vi "Measurement Logic.vi"(8 "error in":errorcluster, 9 "measurement configuration":T2={"TDMS File Location"="", "Run Action"="Create/Replace Wfm Group", "Wfm Group Name"="Wfm1", "Channel Names"=[], "Waveforms Summary JSON"=[]}, 10 "measure call context in":refnum<class "Measure Call Context.lvclass">) -> (0 "error out":errorcluster, 1 "measurement results":T1={"Final Waveform Group Name"="Empty"}, 2 "measure call context out":refnum<class "Measure Call Context.lvclass">)   [LabVIEW 2025, in "TDMS Waveform Creator.lvclass"]
doc: "Contains the core logic for executing the measurement."
uses:
  TDMS Waveform Creator.lvclass
  TDMS Waveform Creator.lvclass/TDMS Waveform Creator.ctl
  Measurement Results.ctl
  <vilib>/Plug-In SDKs/Measurements/Measure Call Context/Measure Call Context.lvclass
  Measurement Configuration.ctl
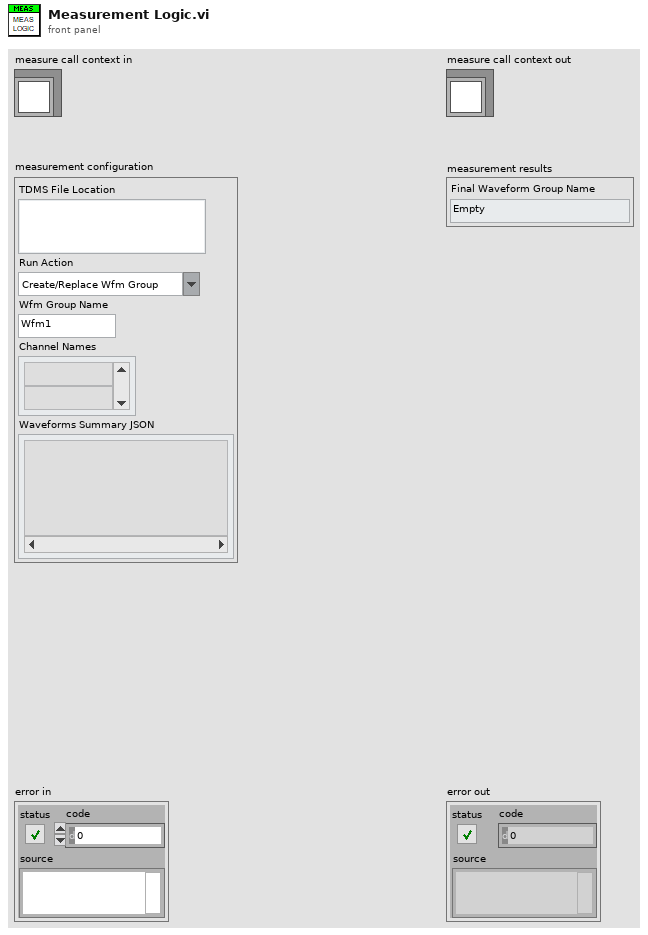
[diagram p1: front panel]
types:
  T1 = typedef "TDMS Waveform Creator.lvclass/Measurement Results.ctl" = cluster{"Final Waveform Group Name":string}
  T2 = typedef "TDMS Waveform Creator.lvclass/Measurement Configuration.ctl" = cluster{"TDMS File Location":string, "Run Action":string, "Wfm Group Name":string, "Channel Names":string[], "Waveforms Summary JSON":string[]}
  T3 = typedef "Event Messenger-bool.lvlib/))Channel.ctl" = refnum<queue>
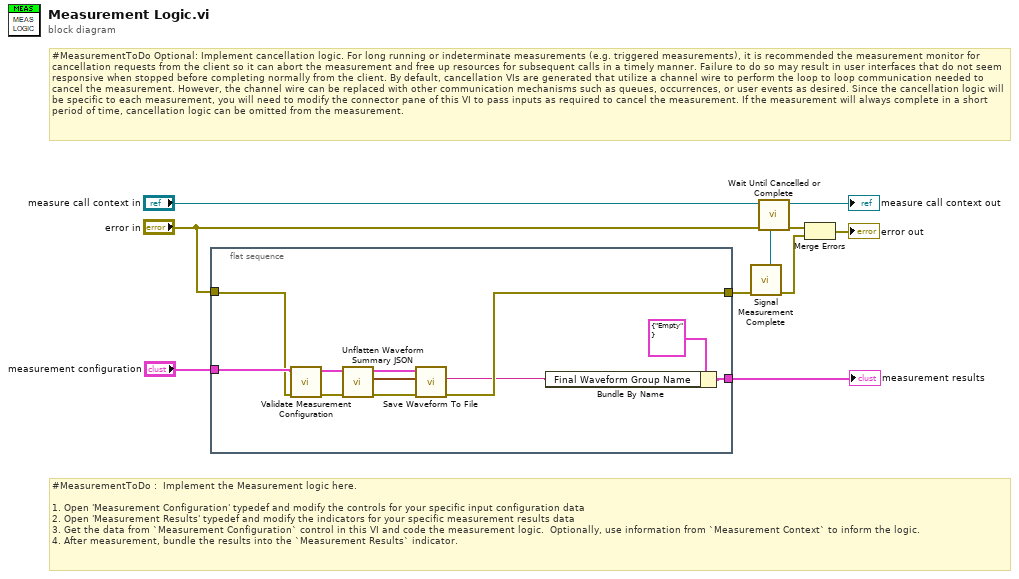
[diagram p0: block diagram]
diagram:
  # "#MeasurementToDo Optional: Implement cancellation logic. For long running or indeterminate measurements (e.g. triggered measurements), it is recommended the measurement monitor for cancellation requests from the client so it can abort the measurement and free up resources for subsequent calls in a timely manner. Failure to do so may result in user interfaces that do not seem responsive when stopped before completing normally from the client. By default, cancellation VIs are generated that utilize a channel wire to perform the loop to loop communication needed to cancel the measurement. However, the channel wire can be replaced with other communication mechanisms such as queues, occurrences, or user events as desired. Since the cancellation logic will be specific to each measurement, you will need to modify the connector pane of this VI to pass inputs as required to cancel the measurement. If the measurement will always complete in a short period of time, cancellation logic can be omitted from the measurement."
  # "#MeasurementToDo :  Implement the Measurement logic here.\n\n1. Open 'Measurement Configuration' typedef and modify the controls for your specific input configuration data\n2. Open 'Measurement Results' typedef and modify the indicators for your specific measurement results data\n3. Get the data from `Measurement Configuration` control in this VI and code the measurement logic.  Optionally, use information from `Measurement Context` to inform the logic.\n4. After measurement, bundle the results into the `Measurement Results` indicator."
  n1 = flat-sequence {
    tunnel: "measurement configuration" -> [w19]
    tunnel: [w20] -> w9
    tunnel: "error in" -> [w17]
    tunnel: [w14] -> w5
    frame #0 {
      n2 = call "Validate Measurement Configuration.vi"("error in"=w17, "Measurement Configuration In"=w19) -> ("error out"=w18:errorcluster, "Measurement Configuration Out"=w15:T2)  [unwired: 8 in]
      n3 = call "Unflatten Waveform Summary JSON.vi"("error in"=w18, "Measurement Configuration In"=w15) -> ("error out"=w16:errorcluster, "Waveforms"=w11:waveform(dbl)[], "Measurement Configuration Out"=w13:T2)  [unwired: 7 in]
      n4 = call "Save Waveform To File.vi"("error in"=w16, "Waveforms"=w11, "Measurement Configuration In"=w13) -> ("error out"=w14:errorcluster, "Final Wfm Group Name"=w12:string)  [unwired: 6 in, 1 out]
      n5 = Bundle By Name(cluster=T1 {"Final Waveform Group Name"="Empty"} ("Measurement Results"), "Final Waveform Group Name"=w12) -> (w20:T1)
    }
  }
  n6 = call "Signal Measurement Complete.vi"("error in (no error)"=w5) -> ("error out"=w3:errorcluster, "done channel"=w4:T3)  [unwired: 9 in]
  n7 = call "Wait Until Cancelled or Complete.vi"("done channel"=w4, "error in (no error)"="error in", "measure call context in"="measure call context in") -> ("error out"=w2:errorcluster, "measure call context out"=→"measure call context out":refnum<class "Measure Call Context.lvclass">)  [unwired: 7 in]
  n8 = Merge Errors(w2, w3) -> (→"error out":errorcluster)
  "measurement results" <- w9
